vi "Get Dirs and Files.vi"(4 "include ..":bool=TRUE, 6 "include .":bool, 8 "error in (no error)":errorcluster, 10 "RemoteDirectory":string, 11 "FTP in":refnum<class "FTP.lvclass">) -> (0 "error out":errorcluster, 1 "Dirs":string[](array[string]), 2 "Files":string[](array[string]), 3 "FTP out":refnum<class "FTP.lvclass">)   [LabVIEW 2017, in "FTP_UpgradeCSMF.lvlib" / "FTP.lvclass"]
uses:
  FTP.lvclass
  controls/Dir-File Type.ctl
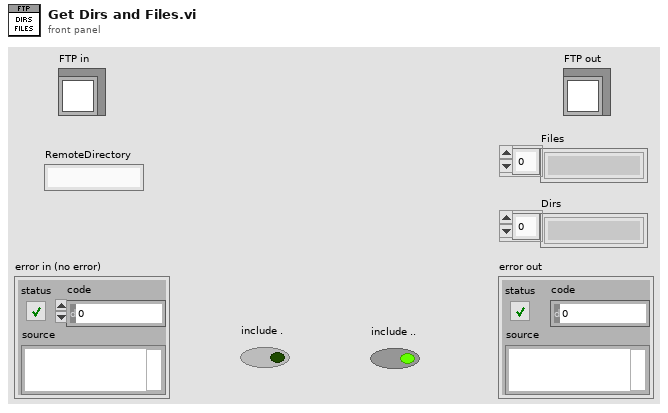
[diagram p1: front panel]
types:
  T1 = typedef "FTP_UpgradeCSMF.lvlib/FTP.lvclass/Dir-File Type.ctl" = enum16{"File", "Listed Directory", "Parent Directory", "Directory", "Unknown"}
  T2 = typedef "FTP_UpgradeCSMF.lvlib/FTP.lvclass/Dir-File Info.ctl" = cluster{"Name":string, "Modify Timestamp":timestamp, "Dir-File Type":T1, "Unique Id":string, "Permissions":string, "Unix Mode":u16, "Owner":string, "Group":string, "FileSize":i64}
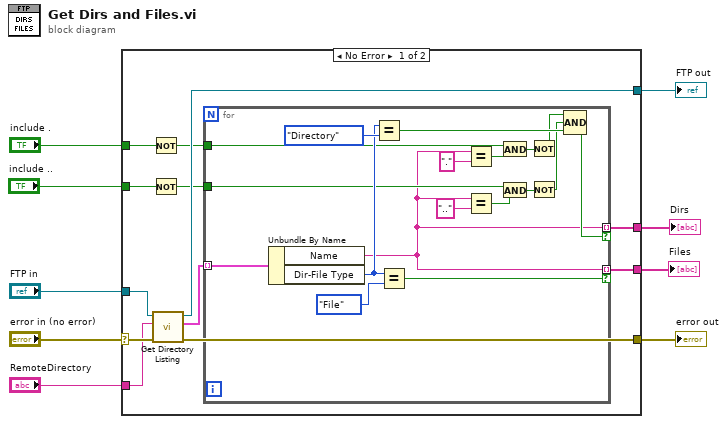
[diagram p0: block diagram]
diagram:
  n1 = case shown="No Error" "error in (no error)" {
    selector: "error in (no error)" -> [w15 _]
    tunnel: [w21 _] -> w1
    tunnel: [w20 _] -> w2
    tunnel: [w18 _] -> w9
    tunnel: [w17 _] -> w8
    tunnel: "FTP in" -> [w16 _]
    tunnel: "RemoteDirectory" -> [w14 _]
    tunnel: "include ." -> [w13 _]
    tunnel: "include .." -> [w12 _]
    frame No Error {
      n2 = Not(x=w13) -> (.not. x?=w11:bool)
      n3 = Not(x=w12) -> (.not. x?=w10:bool)
      n4 = call "Get Directory Listing.vi"("error in (no error)"=w15, "RemoteDirectory"=w14, "FTP in"=w16) -> ("error out"=w17:errorcluster, "Dir-File Info Array"=w19:T2[], "FTP out"=w18:refnum<class "FTP.lvclass">)  [unwired: 6 in]
      n5 = for {
        tunnel: w19 -> [w39] mode=indexing
        tunnel: [w26] -> w20 mode=indexing if=w33
        tunnel: [w26] -> w21 mode=indexing if=w34
        tunnel: w11 -> [w31]
        tunnel: w10 -> [w27]
        n6 = Unbundle By Name(w39) -> ("Name"=w26:string, "Dir-File Type"=w35:T1)
        n7 = Equal?(x=w35, y=Dir-File_Type."Directory") -> (x = y?=w37:bool)
        n8 = Equal?(x=w35, y=Dir-File_Type."File") -> (x = y?=w34:bool)
        n9 = Equal?(x=w26, y=".") -> (x = y?=w32:bool)
        n10 = Equal?(x=w26, y="..") -> (x = y?=w28:bool)
        n11 = And(x=w31, y=w32) -> (x .and. y?=w24:bool)
        n12 = And(x=w27, y=w28) -> (x .and. y?=w25:bool)
        n13 = Not(x=w24) -> (.not. x?=w23:bool)
        n14 = Not(x=w25) -> (.not. x?=w22:bool)
        n15 = Compound Arithmetic op=AND(w23, w22, w37) -> (w33:bool)
      }
    }
    frame Error {
    }
  }
  "Dirs" <- w2
  "Files" <- w1
  "FTP out" <- w9
  "error out" <- w8
